vi "Camera.setup.vi"(8 "error in":errorcluster, 11 "Camera":T1={"Gate.Delay"=0, "Delay.Step"=0, "Gate.Duration"=150000, "#Accum"=10, "SetpointTemp"=-30, "Last Temp"=6, "Current Temp"=4}) -> (0 "error out":errorcluster, 1 "SetpointTemp":i32, 3 "Camera out":T1={"Gate.Delay"=0, "Delay.Step"=0, "Gate.Duration"=150000, "#Accum"=10, "SetpointTemp"=-30, "Last Temp"=6, "Current Temp"=4})   [LabVIEW 2022 SP3]
uses:
  atmcd32d.llb/FanMode_mode typedef.ctl
  atmcd32d.llb/TriggerMode_mode typedef.ctl
  atmcd32d.llb/AcquisitionMode_mode typedef.ctl
  atmcd32d.llb/ReadMode_mode typedef.ctl
  atmcd32d.llb/GateMode_mode typedef.ctl
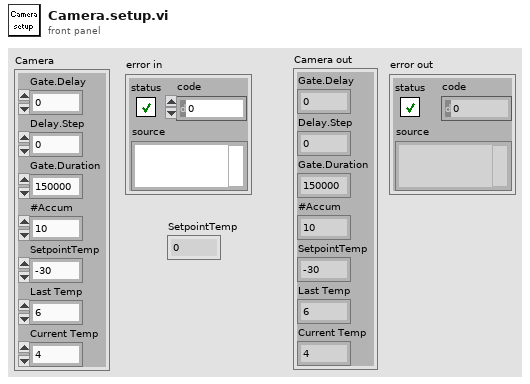
[diagram p1: front panel]
types:
  T1 = cluster{"Gate.Delay":u64, "Delay.Step":u64, "Gate.Duration":u64, "#Accum":i32, "SetpointTemp":i32, "Last Temp":i32, "Current Temp":i32}
  T2 = typedef "GateMode_mode typedef.ctl" = enum16{"Fire ANDed with the Gate input", "Gating controlled from Fire pulse only", "Gating controlled from SMB Gate input only", "Gating ON continuously", "Gating OFF continuously", "Gate using DDG"}
  T3 = typedef "ReadMode_mode typedef.ctl" = enum16{"Full Vertical Binning", "Multi-Track", "Random-Track", "Single-Track", "Image"}
  T4 = typedef "AcquisitionMode_mode typedef.ctl" = enum16{"Reserved (0)", "Single Scan", "Accumulate", "Kinetics", "Fast Kinetics", "Run Till Abort", "Reserved (6)", "Reserved (7)", "Reserved (8)", "Time Delayed Integration"}
  T5 = typedef "TriggerMode_mode typedef.ctl" = enum16{"Internal", "External", "N/A (2)", "N/A (3)", "N/A (4)", "N/A (5)", "External Start", "External Exposure (Bulb)", "N/A (8)", "External FVB EM", "Software", "N/A (11)", "External Charge Shifting"}
  T6 = typedef "FanMode_mode typedef.ctl" = enum16{"fan on full", "fan on low", "fan off"}
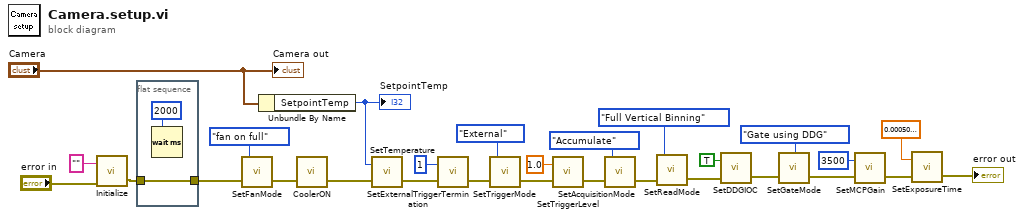
[diagram p0: block diagram]
diagram:
  n1 = call "Initialize.vi"("error in (no error)"="error in", "directory (\"\")"="" ("directory (\"\")")) -> ("error out"=w25:errorcluster)  [unwired: 1 out]
  n2 = flat-sequence {
    tunnel: w25 -> [w29]
    tunnel: [w29] -> w24
    frame #0 {
      n3 = Wait (ms)(milliseconds to wait=u32 2000) -> ()  [unwired: 1 out]
    }
  }
  n4 = call "SetFanMode.vi"("error in (no error)"=w24, "mode"=FanMode_mode_typedef."fan on full") -> ("error out"=w23:errorcluster)  [unwired: 1 out]
  n5 = Unbundle By Name("Camera") -> ("SetpointTemp"=w5:i32)
  "SetpointTemp" <- w5
  n6 = call "CoolerON.vi"("error in (no error)"=w23) -> ("error out"=w22:errorcluster)  [unwired: 1 in, 1 out]
  n7 = call "SetTemperature.vi"("error in (no error)"=w22, "temperature"=w5) -> ("error out"=w20:errorcluster)  [unwired: 1 out]
  n8 = call "SetExternalTriggerTermination.vi"("error in (no error)"=w20, "Termination"=u32 1) -> ("error out"=w18:errorcluster)  [unwired: 1 out]
  n9 = call "SetTriggerMode.vi"("error in (no error)"=w18, "mode"=TriggerMode_mode_typedef."External") -> ("error out"=w17:errorcluster)  [unwired: 1 out]
  n10 = call "SetTriggerLevel.vi"("error in (no error)"=w17, "level"=sgl 1.0) -> ("error out"=w15:errorcluster)  [unwired: 1 out]
  n11 = call "SetAcquisitionMode.vi"("error in (no error)"=w15, "mode"=AcquisitionMode_mode_typedef."Accumulate") -> ("error out"=w12:errorcluster)  [unwired: 1 out]
  n12 = call "SetReadMode.vi"("error in (no error)"=w12, "mode"=ReadMode_mode_typedef."Full Vertical Binning") -> ("error out"=w10:errorcluster)  [unwired: 1 out]
  n13 = call "SetDDGIOC.vi"("error in (no error)"=w10, "integrate"=TRUE) -> ("error out"=w8:errorcluster)  [unwired: 1 out]
  n14 = call "SetGateMode.vi"("error in (no error)"=w8, "mode"=GateMode_mode_typedef."Gate using DDG") -> ("error out"=w7:errorcluster)  [unwired: 1 out]
  n15 = call "SetMCPGain.vi"("error in (no error)"=w7, "gain"=3500) -> ("error out"=w2:errorcluster)  [unwired: 1 out]
  n16 = call "SetExposureTime.vi"("error in (no error)"=w2, "time"=sgl 0.0005) -> ("error out"=→"error out":errorcluster)  [unwired: 1 out]
  "Camera out" <- "Camera"
